vi "newworksheet.vi"   [LabVIEW 2014]
uses:
  <vilib>/Utility/NIReport.llb/Excel/NI_Excel.lvclass
  <vilib>/Utility/NIReport.llb/NI_report.lvclass
types:
  T1 = enum16{"Standard Report", "HTML", "Word", "Excel"}
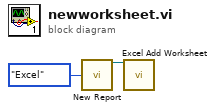
[diagram p0: block diagram]
diagram:
  n1 = call <vilib>:"New Report.vi"("report type"=T1."Excel") -> ("report out"=w1:refnum<class "NI_report.lvclass">)  [unwired: 13 in, 1 out]
  n2 = call <vilib>:"Excel Add Worksheet.vi"("report in"=w1) -> ()  [unwired: 13 in, 2 out]
